vi "Init.vi"(7 "I2C":T2=-1, 8 "error in (no error)":errorcluster, 11 "Address":T1 format="%02x") -> (0 "error out":errorcluster, 3 "I2C Peripheral":refnum<class "I2C Peripheral.lvclass">)   [LabVIEW 2020, in "CTI.lvlib" / "I2C Peripheral.lvclass"]
uses:
  I2C Peripheral.lvclass
  I2C Number.ctl
  I2C Address.ctl
  I2C Peripheral.lvclass/I2C Peripheral.ctl
  CTI.lvlib
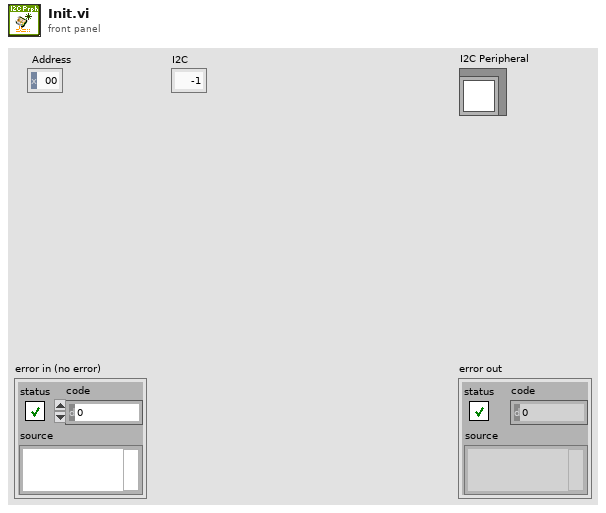
[diagram p1: front panel]
types:
  T1 = typedef "CTI.lvlib/I2C Address.ctl" = u8
  T2 = typedef "CTI.lvlib/I2C Number.ctl" = i8
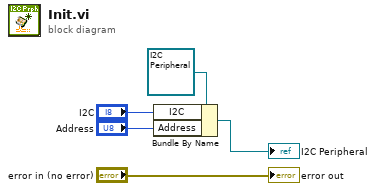
[diagram p0: block diagram]
diagram:
  n1 = Bundle By Name(cluster=refnum<class "I2C Peripheral.lvclass"> refnum ("I2C Device in"), "I2C"="I2C", "Address"="Address") -> (→"I2C Peripheral":refnum<class "I2C Peripheral.lvclass">)
  "error out" <- "error in (no error)"
